vi "Parse.vi"(8 "Error In":errorcluster, 11 "object in":refnum<class "2024_12.lvclass">) -> (0 "Error Out":errorcluster, 3 "object out":refnum<class "2024_12.lvclass">)   [LabVIEW 2023, in "2024_12.lvclass"]
uses:
  2024_12.lvclass
  2024_12.lvclass/2024_12.ctl
  <vilib>/Utility/error.llb/Trim Whitespace One-Sided.vi
  <userlib>/_OpenG.lib/string/string.llb/openg_string.lvlib
panel:
  out "min value":u8
  out "max value":u8
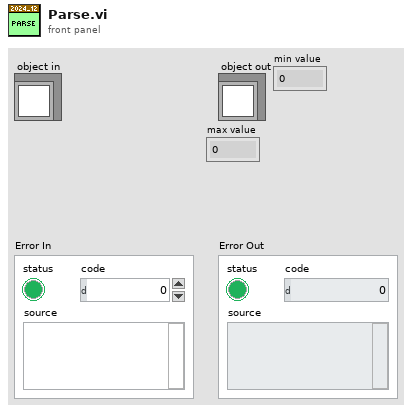
[diagram p1: front panel]
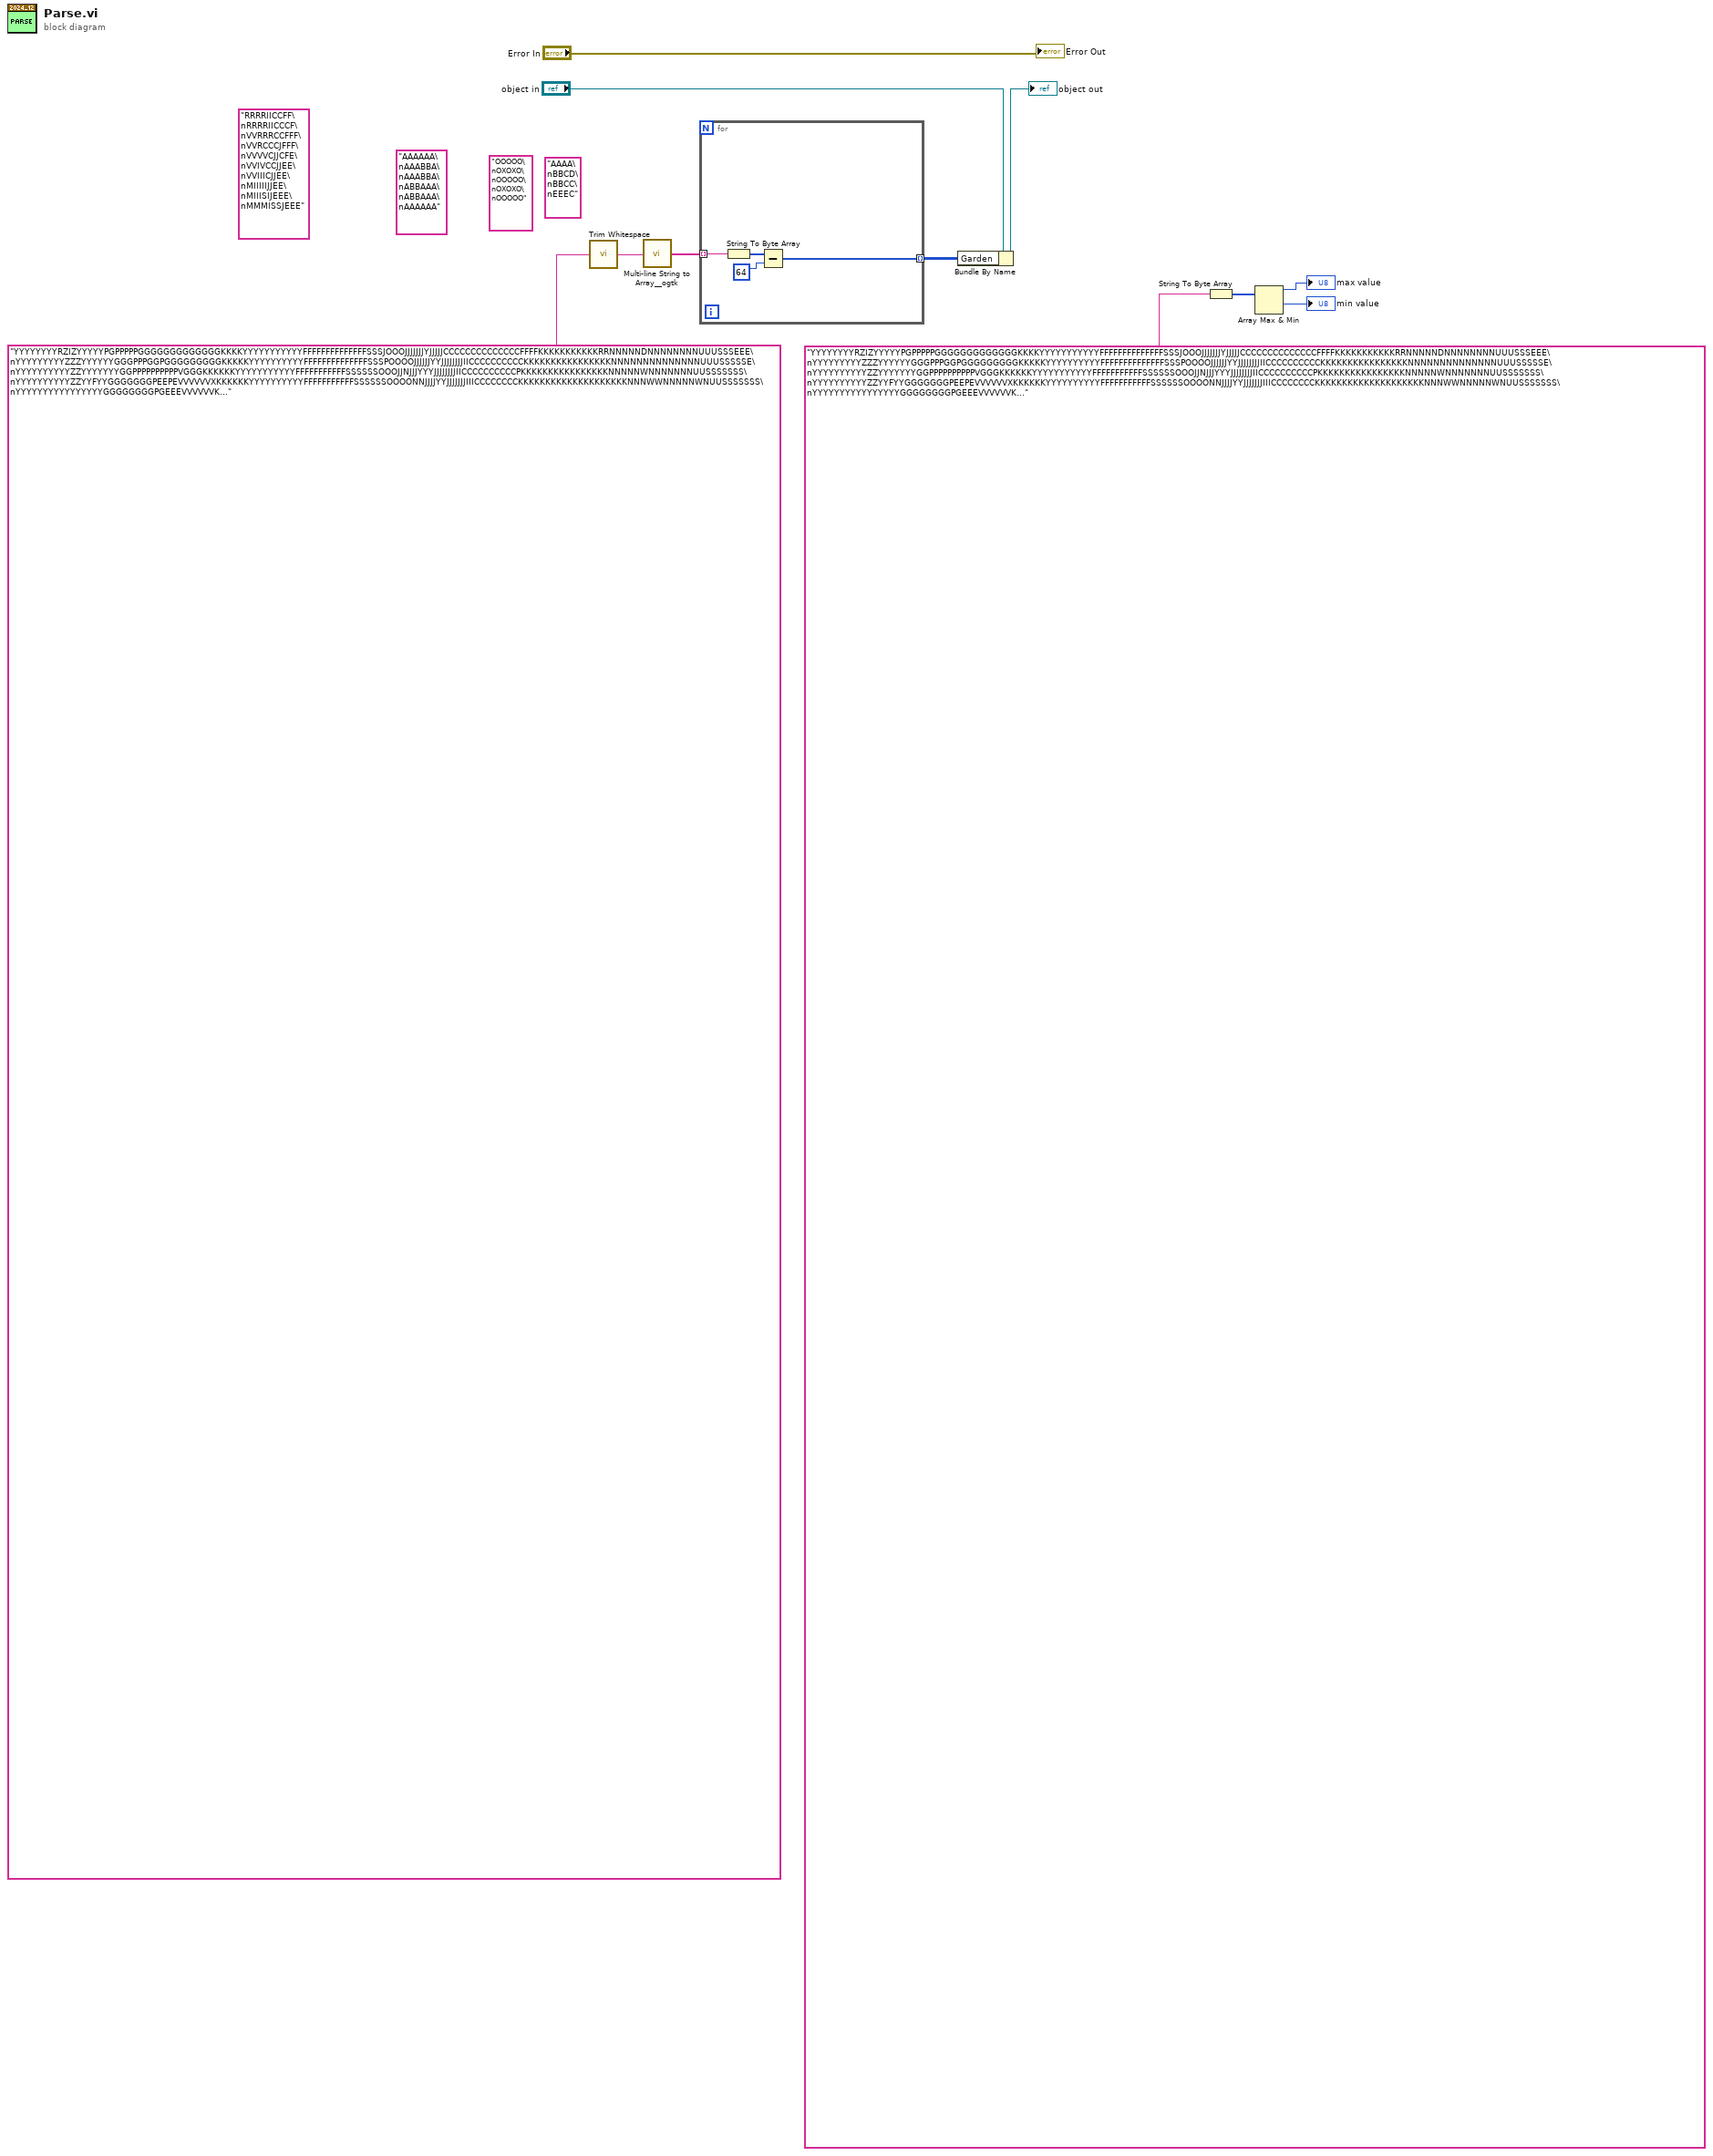
[diagram p0: block diagram]
diagram:
  (unwired) "AAAAAA\nAAABBA\nAAABBA\nABBAAA\nABBAAA\nAAAAAA" ("PuzzleInput")
  (unwired) "RRRRIICCFF\nRRRRIICCCF\nVVRRRCCFFF\nVVRCCCJFFF\nVVVVCJJCFE\nVVIVCCJJEE\nVVIIICJJEE\nMIIIIIJJEE\nMIIISIJEEE\nMMMISSJEEE" ("PuzzleInput")
  (unwired) "OOOOO\nOXOXO\nOOOOO\nOXOXO\nOOOOO" ("PuzzleInput")
  (unwired) "AAAA\nBBCD\nBBCC\nEEEC" ("PuzzleInput")
  n1 = call <vilib>:"Trim Whitespace.vi"("string"="YYYYYYYYRZIZYYYYYPGPPPPPGGGGGGGGGGGGGKKKKYYYYYYYYYYYFFFFFFFFFFFFFFSSSJOOOJJJJJJJYJJJJJCCCCCCCCCCCCCCFFFFKKKKKKKKKKKRRNNNNNDNNNNNNNNUUUSSSEEE\nYYYYYYYYYZZZYYYYYYGGGPPPGGPGGGGGGGGGKKKKKYYYYYYYYYYFFFFFFFFFFFFFFSSSPOOOOJJJJJJYYJJJJJJJJIICCCCCCCCCCKKKKKKKKKKKKKKKKNNNNNNNNNNNNNNUUUSSSSSE\nYYYYYYYYYYZZYYYYYYYGGPPPPPPPPPPVGGGKKKKKKYYYYYYYYYYYFFFFFFFFFFFSSSSSSOOOJJNJJJYYYJJJJJJJJIICCCCCCCCCCPKKKKKKKKKKKKKKKKNNNNNWNNNNNNNUUSSSSSSS\nYYYYYYYYYYZZYYFYYGGGGGGGPEEPEVVVVVVXKKKKKKYYYYYYYYYYFFFFFFFFFFFSSSSSSOOOONNJJJJYYJJJJJJJIIICCCCCCCCKKKKKKKKKKKKKKKKKKKKNNNWWNNNNNWNUUSSSSSSS\nYYYYYYYYYYYYYYYYGGGGGGGGPGEEEVVVVVVK..." ("PuzzleInput")) -> ("trimmed string"=w8:string)  [unwired: 1 in]
  n2 = call <userlib>:"Multi-line String to Array__ogtk.vi"("string"=w8) -> ("lines"=w7:string[])
  n3 = for {
    tunnel: w7 -> [w15] mode=indexing
    tunnel: [w12] -> w6 mode=indexing
    n4 = String To Byte Array(string=w15) -> (unsigned byte array=w14:u8[])
    n5 = Subtract(x=w14, y=u8 64) -> (x-y=w12:u8[])
  }
  n6 = Bundle By Name(cluster="object in", "Garden"=w6) -> (→"object out":refnum<class "2024_12.lvclass">)
  n7 = String To Byte Array(string="YYYYYYYYRZIZYYYYYPGPPPPPGGGGGGGGGGGGGKKKKYYYYYYYYYYYFFFFFFFFFFFFFFSSSJOOOJJJJJJJYJJJJJCCCCCCCCCCCCCCFFFFKKKKKKKKKKKRRNNNNNDNNNNNNNNUUUSSSEEE\nYYYYYYYYYZZZYYYYYYGGGPPPGGPGGGGGGGGGKKKKKYYYYYYYYYYFFFFFFFFFFFFFFSSSPOOOOJJJJJJYYJJJJJJJJIICCCCCCCCCCKKKKKKKKKKKKKKKKNNNNNNNNNNNNNNUUUSSSSSE\nYYYYYYYYYYZZYYYYYYYGGPPPPPPPPPPVGGGKKKKKKYYYYYYYYYYYFFFFFFFFFFFSSSSSSOOOJJNJJJYYYJJJJJJJJIICCCCCCCCCCPKKKKKKKKKKKKKKKKNNNNNWNNNNNNNUUSSSSSSS\nYYYYYYYYYYZZYYFYYGGGGGGGPEEPEVVVVVVXKKKKKKYYYYYYYYYYFFFFFFFFFFFSSSSSSOOOONNJJJJYYJJJJJJJIIICCCCCCCCKKKKKKKKKKKKKKKKKKKKNNNWWNNNNNWNUUSSSSSSS\nYYYYYYYYYYYYYYYYGGGGGGGGPGEEEVVVVVVK..." ("PuzzleInput")) -> (unsigned byte array=w4:u8[])
  n8 = Array Max & Min(array=w4) -> (max value=→"max value":u8, min value=→"min value":u8)  [unwired: 2 out]
  "Error Out" <- "Error In"
